vi "Spont1.vi"() -> ()   [LabVIEW 2013]
uses:
  <vilib>/Utility/file.llb/Write To Spreadsheet File (DBL).vi
panel:
  out "delta_counts":dbl=0.047057108471881826
  out "cursor y":dbl=1.0022428708747197
  out "Intensity Graph":u16[][](graph)
  out "transposed array":u16[][](array[numeric])
  in  "focus":bool
  in  "Filename":string="test"
  in  "SetPath":bool
  in  "Path":string="C:\\data"
  in  "Acquire 2":bool
  in  "Number of acquisitions":dbl=10.0 format="%.3f"
  in  "Acquire":bool
  out "Temperature":dbl=-75.0
  in  "stop":bool
  in  "Save?":bool
  out "Waveform Graph":dbl[](graph)
  in  "Exposure Time (s)":dbl=1.0 format="%.3f"
  out "error out":errorcluster
  in  "error in (no error)":errorcluster
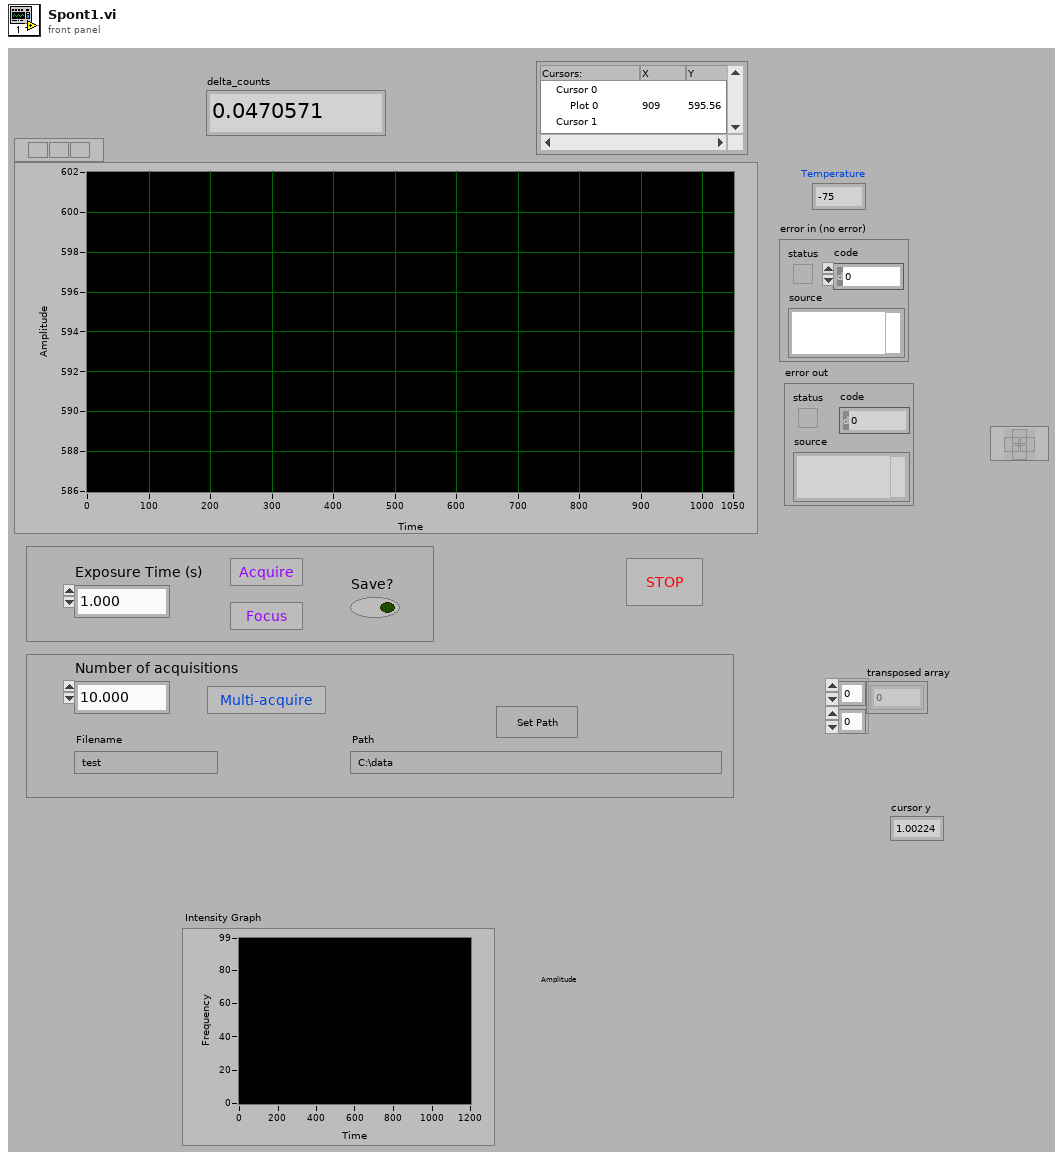
[diagram p1: front panel]
types:
  T1 = cluster{"Camera Handle":u32, "File Handle":u32, "Image Handle":u32}
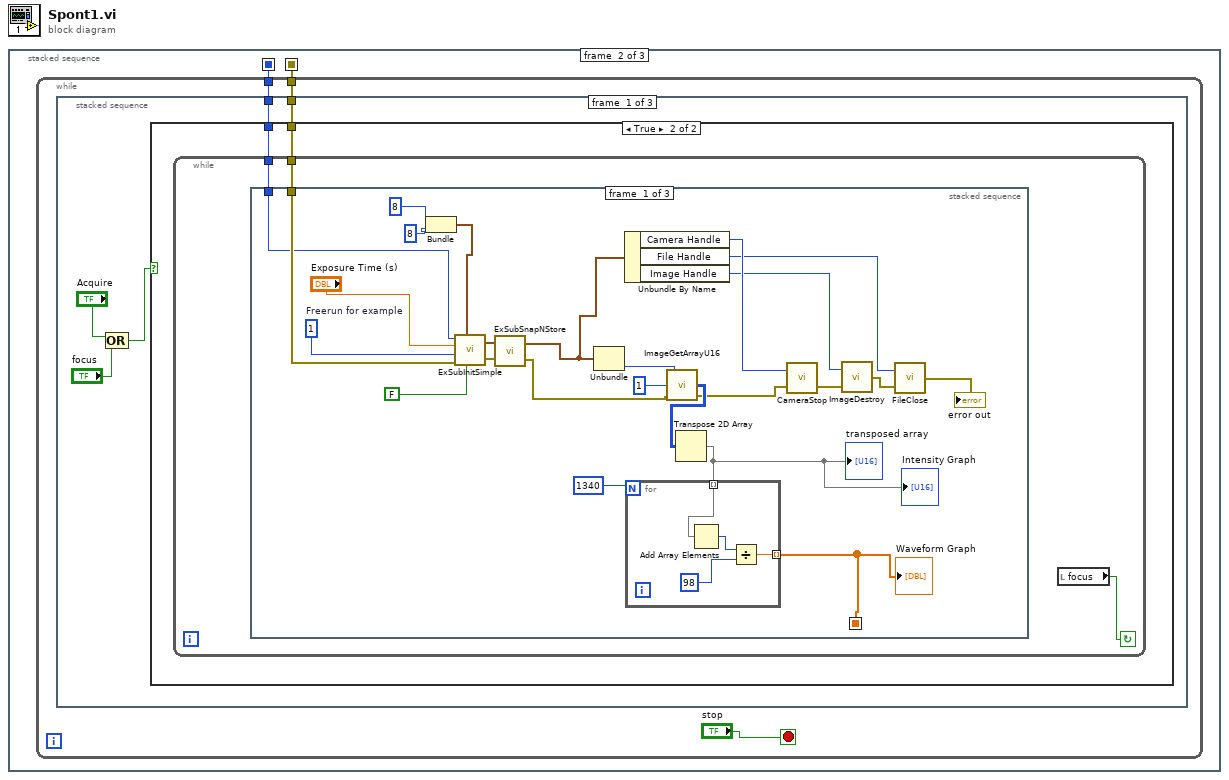
[diagram p0: block diagram]
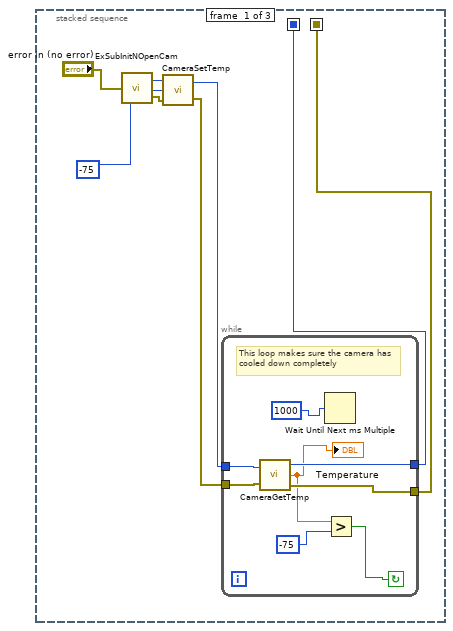
[diagram p2: hidden frame]
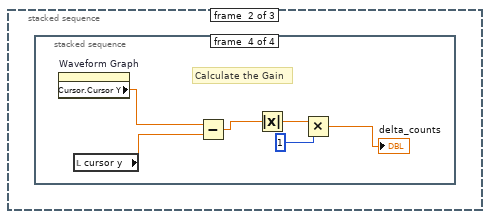
[diagram p4: hidden frame]
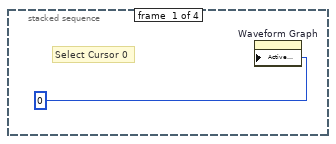
[diagram p5: hidden frame]
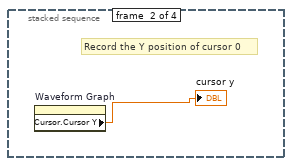
[diagram p6: hidden frame]
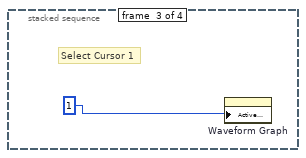
[diagram p7: hidden frame]
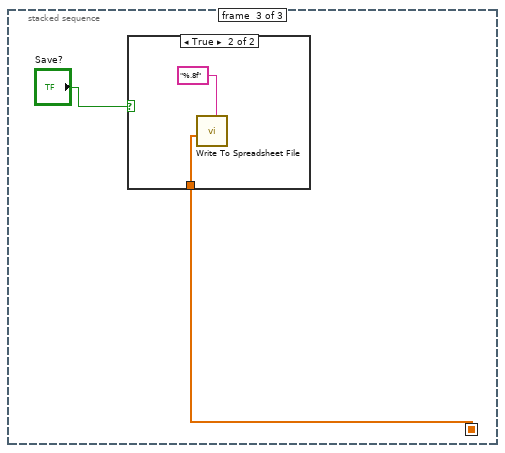
[diagram p8: hidden frame]
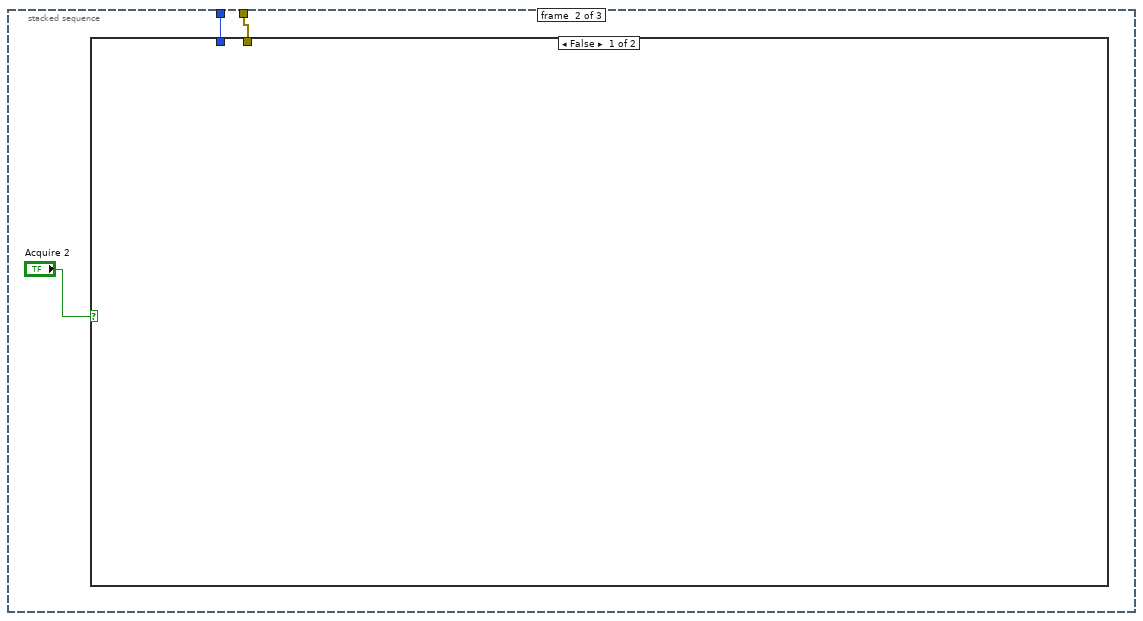
[diagram p10: hidden frame]
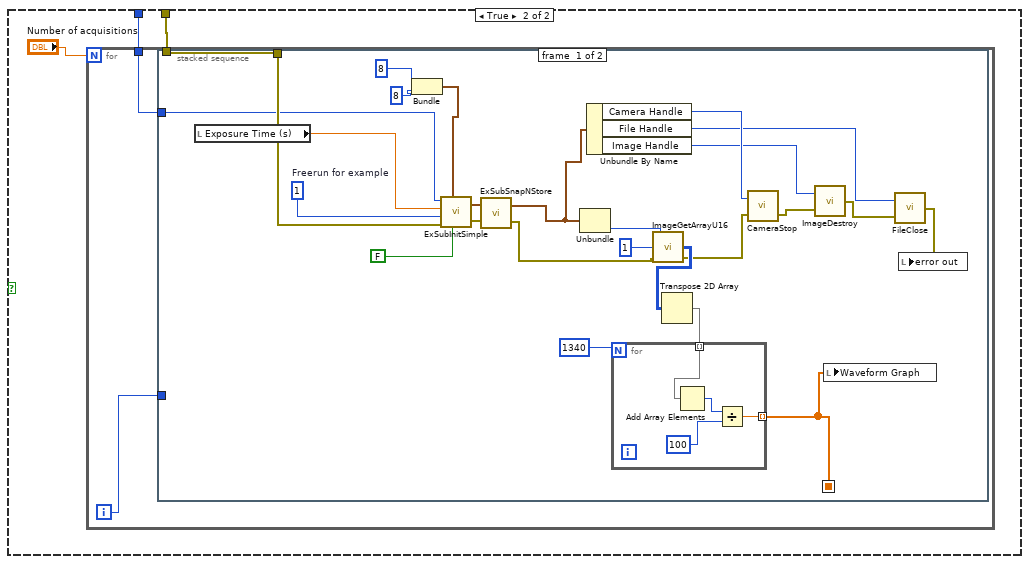
[diagram p11: hidden frame]
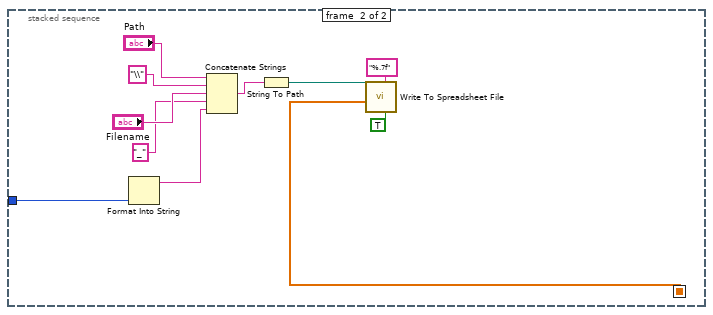
[diagram p12: hidden frame]
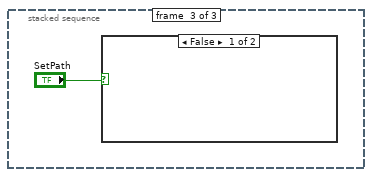
[diagram p13: hidden frame]
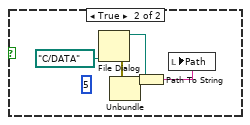
[diagram p14: hidden frame]
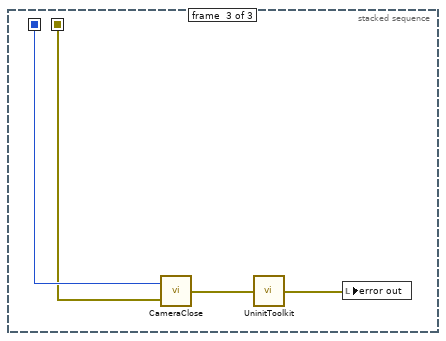
[diagram p15: hidden frame]
diagram:
  n1 = stacked-sequence {
    seq-local: [w2 _ _] -> [_ w18 w130]
    seq-local: [w1 _ _] -> [_ w17 w131]
    frame #0 {
      n2 = call "ExSubInitNOpenCam.vi"("error in (no error)"="error in (no error)") -> ("Camera Handle"=w5:u32, "error out"=w7:errorcluster)
      n3 = call <userlib>:"CameraSetTemp.vi"("error in (no error)"=w7, "Temperature"=-75, "Camera Handle"=w5) -> ("error out"=w3:errorcluster, "Camera Handle"=w4:u32)
      n4 = while {
        tunnel: w3 -> [w15]
        tunnel: [w14] -> w2
        tunnel: w4 -> [w13]
        tunnel: [w12] -> w1
        stop <- w10 continue-if-true
        # "This loop makes sure the camera has cooled down completely"
        n5 = call <userlib>:"CameraGetTemp.vi"("Camera Handle"=w13, "error in (no error)"=w15) -> ("Camera Handle"=w12:u32, "Temperature"=w9:dbl, "error out"=w14:errorcluster)
        "Temperature" <- w9
        n6 = Wait Until Next ms Multiple(millisecond multiple=1000 ("ADC Gain")) -> ()  [unwired: 1 out]
        n7 = Greater?(x=w9, y=-75) -> (0:w10:bool)
      }
    }
    frame #1 {
      n8 = while {
        tunnel: w18 -> [w20]
        tunnel: w17 -> [w19]
        stop <- "stop" stop-if-true
        n9 = stacked-sequence {
          tunnel: w20 -> [w26 w75 _]
          tunnel: w19 -> [w25 w74 _]
          frame #0 {
            n10 = Compound Arithmetic op=OR("Acquire", "focus") -> (w22:bool)
            n11 = case shown="True" w22 {
              tunnel: w26 -> [_ w28]
              tunnel: w25 -> [_ w27]
              frame False {
              }
              frame True {
                n12 = while {
                  tunnel: w28 -> [w31]
                  tunnel: w27 -> [w30]
                  stop <- w29 continue-if-true
                  n13 = stacked-sequence {
                    seq-local: [w43 _ _] -> [_ _ w70]
                    tunnel: w31 -> [w42 _ _]
                    tunnel: w30 -> [w41 _ _]
                    frame #0 {
                      w54 = 1  # Freerun for example
                      n14 = Bundle(8, 8) -> (w52:cluster{i32, i32})  [unwired: 1 in]
                      n15 = call "ExSubInitSimple.vi"("Intensifier"=FALSE, "Shutter Comp"=w52, "error in (no error)"=w42, "Triggering mode"=w54, "Exposure"="Exposure Time (s)", "Camera Handle"=w41) -> ("error out"=w51:errorcluster, "Handles"=w50:cluster{"Camera":u32, "File":u32, "Image":u32})
                      n16 = call "ExSubSnapNStore.vi"("error in (no error)"=w51, "Handle Cluster"=w50) -> ("error out"=w46:errorcluster, "Handle Cluster Out"=w40:T1)
                      n17 = Unbundle(w40) -> ("Image Handle"=w47:u32)  [unwired: 2 out]
                      n18 = Unbundle By Name(w40) -> ("Camera Handle"=w39:u32, "File Handle"=w38:u32, "Image Handle"=w35:u32)
                      n19 = call <userlib>:"ImageGetArrayU16.vi"("error in"=w46, "Z position"=1, "Image Handle"=w47) -> ("error out"=w37:errorcluster, "Array uint 16"=w45:u16[][])  [unwired: 1 out]
                      n20 = Transpose 2D Array(2D array=w45) -> (transposed array=w32:u16[][])
                      "transposed array" <- w32
                      "Intensity Graph" <- w32
                      n21 = for {
                        N: 1340 -> [_]
                        tunnel: w32 -> [w60] mode=indexing
                        tunnel: [w57] -> w43 mode=indexing
                        n22 = Add Array Elements(numeric array=w60) -> (sum=w59:u16)
                        n23 = Divide(x=w59, y=98) -> (x/y=w57:dbl)
                      }
                      "Waveform Graph" <- w43
                      n24 = call <userlib>:"CameraStop.vi"("error in"=w37, "Camera Handle"=w39) -> ("error out"=w34:errorcluster)  [unwired: 1 out]
                      n25 = call <userlib>:"ImageDestroy.vi"("error in"=w34, "Data handle"=w35) -> ("error out"=w33:errorcluster)
                      n26 = call <userlib>:"FileClose.vi"("error in"=w33, "File Handle"=w38) -> ("error out"=→"error out":errorcluster)
                    }
                    frame #1 {
                      n27 = stacked-sequence {
                        frame #0 {
                          # "Select Cursor 0"
                          n28 = property on="Waveform Graph" class="WFGraph (strict)"("Active Cursor"=0) -> ()  [unwired: 2 in, 2 out]
                        }
                        frame #1 {
                          # "Record the Y position of cursor 0"
                          n29 = property on="Waveform Graph" class="WFGraph (strict)"() -> ("Cursor.Cursor Y"=→"cursor y":dbl)  [unwired: 2 in, 2 out]
                        }
                        frame #2 {
                          # "Select Cursor 1"
                          n30 = property on="Waveform Graph" class="WFGraph (strict)"("Active Cursor"=1) -> ()  [unwired: 2 in, 2 out]
                        }
                        frame #3 {
                          # "Calculate the Gain"
                          n31 = property on="Waveform Graph" class="WFGraph (strict)"() -> ("Cursor.Cursor Y"=w64:dbl)  [unwired: 2 in, 2 out]
                          n32 = local read "cursor y"() -> (w69:dbl)
                          n33 = Subtract(x=w64, y=w69) -> (x-y=w66:dbl)
                          n34 = Absolute Value(x=w66) -> (abs(x)=w68:dbl)
                          n35 = Multiply(x=w68, y=1) -> (x*y=→"delta_counts":dbl)
                        }
                      }
                    }
                    frame #2 {
                      n36 = case shown="True" "Save?" {
                        tunnel: w70 -> [_ w72]
                        frame False {
                        }
                        frame True {
                          n37 = call-poly <vilib>:"Write To Spreadsheet File.vi"("format (%.3f)"="%.8f", "1D data"=w72) -> ()  [unwired: 6 in, 1 out]
                        }
                      }
                    }
                  }
                  n38 = local read "focus"() -> (w29:bool)
                }
              }
            }
          }
          frame #1 {
            n39 = case shown="False" "Acquire 2" {
              tunnel: w75 -> [_ w78]
              tunnel: w74 -> [_ w77]
              frame False {
              }
              frame True {
                n40 = for {
                  N: "Number of acquisitions" -> [_]
                  tunnel: w78 -> [w81]
                  tunnel: w77 -> [w80]
                  i -> [w82]
                  n41 = stacked-sequence {
                    seq-local: [w91 _] -> [_ w112]
                    tunnel: w82 -> [_ w122]
                    tunnel: w81 -> [w94 _]
                    tunnel: w80 -> [w93 _]
                    frame #0 {
                      w105 = 1  # Freerun for example
                      n42 = local read "Exposure Time (s)"() -> (w92:dbl)
                      n43 = Bundle(8, 8) -> (w104:cluster{i32, i32})  [unwired: 1 in]
                      n44 = call "ExSubInitSimple.vi"("Intensifier"=FALSE, "Shutter Comp"=w104, "error in (no error)"=w94, "Triggering mode"=w105, "Exposure"=w92, "Camera Handle"=w93) -> ("error out"=w103:errorcluster, "Handles"=w102:cluster{"Camera":u32, "File":u32, "Image":u32})
                      n45 = call "ExSubSnapNStore.vi"("error in (no error)"=w103, "Handle Cluster"=w102) -> ("error out"=w98:errorcluster, "Handle Cluster Out"=w88:T1)
                      n46 = Unbundle(w88) -> ("Image Handle"=w99:u32)  [unwired: 2 out]
                      n47 = Unbundle By Name(w88) -> ("Camera Handle"=w90:u32, "File Handle"=w89:u32, "Image Handle"=w84:u32)
                      n48 = call <userlib>:"ImageGetArrayU16.vi"("error in"=w98, "Z position"=1, "Image Handle"=w99) -> ("error out"=w87:errorcluster, "Array uint 16"=w97:u16[][])  [unwired: 1 out]
                      n49 = Transpose 2D Array(2D array=w97) -> (transposed array=w95:u16[][])
                      n50 = for {
                        N: 1340 -> [_]
                        tunnel: w95 -> [w111] mode=indexing
                        tunnel: [w108] -> w91 mode=indexing
                        n51 = Add Array Elements(numeric array=w111) -> (sum=w110:u16)
                        n52 = Divide(x=w110, y=100) -> (x/y=w108:dbl)
                      }
                      n53 = call <userlib>:"CameraStop.vi"("error in"=w87, "Camera Handle"=w90) -> ("error out"=w85:errorcluster)  [unwired: 1 out]
                      n54 = call <userlib>:"ImageDestroy.vi"("error in"=w85, "Data handle"=w84) -> ("error out"=w83:errorcluster)
                      n55 = local write "Waveform Graph"(w91) -> ()
                      n56 = call <userlib>:"FileClose.vi"("error in"=w83, "File Handle"=w89) -> ("error out"=w86:errorcluster)
                      n57 = local write "error out"(w86) -> ()
                    }
                    frame #1 {
                      n58 = Format Into String(w122) -> (resulting string=w117:string)  [unwired: 3 in, 1 out]
                      n59 = Concatenate Strings("Path", "\\", "Filename", "_", w117) -> (w116:string)
                      n60 = String To Path(string=w116) -> (path=w113:path)
                      n61 = call-poly <vilib>:"Write To Spreadsheet File.vi"("transpose? (no:F)"=TRUE, "format (%.3f)"="%.7f", "1D data"=w112, "file path (dialog if empty)"=w113) -> ()  [unwired: 4 in, 1 out]
                    }
                  }
                }
              }
            }
          }
          frame #2 {
            n62 = case shown="False" "SetPath" {
              frame False {
              }
              frame True {
                (unwired) 5
                n63 = File Dialog(11:path "C:/DATA") -> (0:w124:errorcluster, 3:w127:path)  [unwired: 6 in, 2 out]
                n64 = Unbundle(w124) -> ()  [unwired: 3 out]
                n65 = Path To String(path=w127) -> (string=w125:string)
                n66 = local write "Path"(w125) -> ()
              }
            }
          }
        }
      }
    }
    frame #2 {
      n67 = call <userlib>:"CameraClose.vi"("error in"=w130, "Camera Handle"=w131) -> ("error out"=w129:errorcluster)
      n68 = call <userlib>:"UninitToolkit.vi"("error in"=w129) -> ("error out"=w128:errorcluster)
      n69 = local write "error out"(w128) -> ()
    }
  }
